vi "Cmd.HandleErrorMsg.vi"(1 "Response":string) -> (8 "ErrorMsg":string)   [LabVIEW 2016]
uses:
  controls/Command.ctl
panel:
  in  "Command":T1=[{"Cmd"="Trigger 1", "CmdShortcut"="T1"}, {"Cmd"="Switch to run mode", "CmdShortcut"="R0"}, {"Cmd"="unknown", "CmdShortcut"="xx"}]
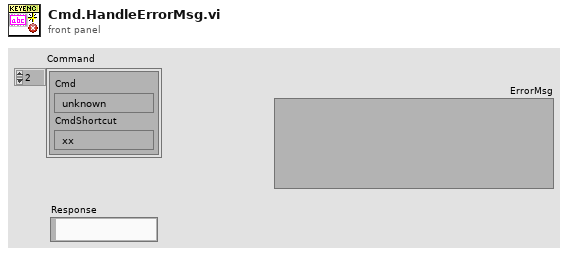
[diagram p1: front panel]
types:
  T1 = typedef "Command.ctl" = cluster{"Cmd":string, "CmdShortcut":string}[]
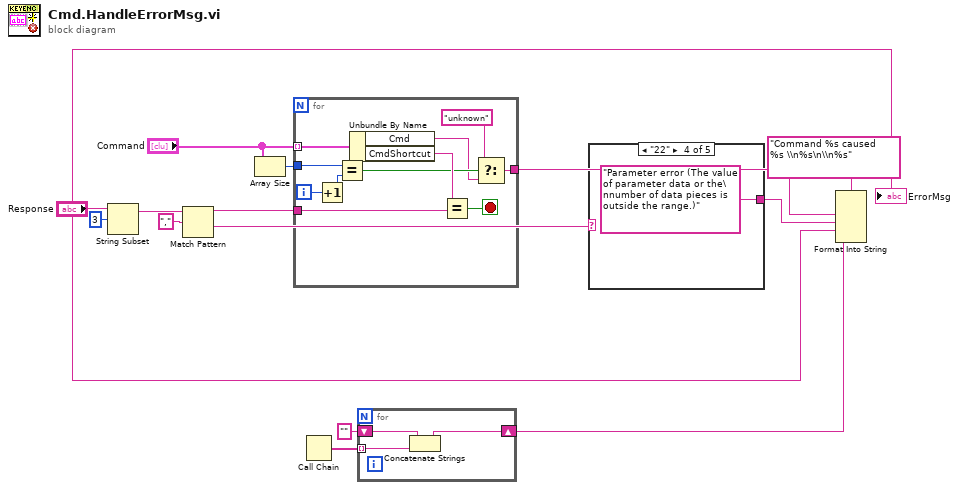
[diagram p0: block diagram]
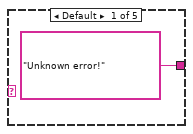
[diagram p2: hidden frame]
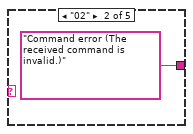
[diagram p3: hidden frame]
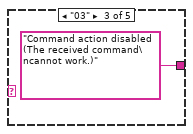
[diagram p4: hidden frame]
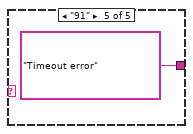
[diagram p5: hidden frame]
diagram:
  n1 = String Subset(string="Response", offset (0)=3) -> (substring=w7:string)  [unwired: 1 in]
  n2 = Match Pattern(string=w7, regular expression=",") -> (before substring=w13:string, after substring=w12:string)  [unwired: 1 in, 2 out]
  n3 = Array Size(array="Command") -> (size(s)=w6:i32)
  n4 = for {
    tunnel: "Command" -> [w25] mode=indexing
    tunnel: w13 -> [w24]
    tunnel: [w17] -> w9
    tunnel: w6 -> [w21]
    i -> [w16]
    stop <- w22 stop-if-true
    n5 = Increment(x=w16) -> (x+1=w15:i32)
    n6 = Equal?(x=w21, y=w15) -> (x = y?=w20:bool)
    n7 = Unbundle By Name(w25) -> ("Cmd"=w19:string, "CmdShortcut"=w23:string)
    n8 = Equal?(x=w23, y=w24) -> (x = y?=w22:bool)
    n9 = Select(t="unknown", s=w20, f=w19) -> (s? t:f=w17:string)
  }
  n10 = Call Chain() -> (call chain=w4:string[])
  n11 = for {
    tunnel: w4 -> [w28] mode=indexing
    shift-right: [w26] -> w2
    shift-left: "" -> [w27]
    n12 = Concatenate Strings(w27, w28) -> (w26:string)
  }
  n13 = case shown="\"22\"" w12 {
    tunnel: ["Unknown error!" "Command error (The received command is invalid.)" "Command action disabled (The received command\ncannot work.)" "Parameter error (The value of parameter data or the\nnumber of data pieces is outside the range.)" "Timeout error"] -> w10
    frame Default {
    }
    frame "02" {
    }
    frame "03" {
    }
    frame "22" {
    }
    frame "91" {
    }
  }
  n14 = Format Into String(format string="Command %s caused %s \\n%s\n\\n%s", w9, w10, "Response", w2) -> ()  [unwired: 2 in, 2 out]
  "ErrorMsg" <- "Response"
